vi "Main.vi"(7 "sweep rate, /min":dbl=0.2, 8 "sweep to:":dbl=-0.5, 9 "sweep":T3(radio)=enum."time_sweep") -> ()   [LabVIEW 2017] (continued)
                          tunnel: w368 -> [w372 w376]
                          tunnel: [w372 w374] -> w367
                          frame False {
                            # "not measure SR830 3 out of phase signal (SR830_3_oop)"
                          }
                          frame True {
                            w375 = "SR830_3_oop"
                            # "measure SR830 3 out phase signal (SR830_3_oop)"
                            n376 = local read "SR830 3 addr"() -> (w380:u8)
                            n377 = Number To Decimal String(number=w380) -> (decimal integer string=w381:string)  [unwired: 1 in]
                            n378 = GPIB Clear(3:w381) -> ()  [unwired: 1 in, 2 out]
                            n379 = Build Array (concatenate)(w376, w375) -> (w374:string[])
                            n380 = Concatenate Strings(w379, w375, "\t") -> (w378:string)
                          }
                        }
                        n381 = property on="Figure_axis" class="Arr (strict)"("Value"=w367) -> ()  [unwired: 2 in, 2 out]
                        n382 = property on="data_caption" class="Str"("Value"=w369) -> ()  [unwired: 2 in, 2 out]
                      }
                      frame #6 {
                        # "SR830 4 in phase (SR830_4_ip)"
                        n383 = local read "SR830 4 ip"() -> (w386:bool)
                        n384 = property on="Figure_axis" class="Arr (strict)"() -> ("Value"=w383:string[])  [unwired: 2 in, 2 out]
                        n385 = property on="data_caption" class="Str"() -> ("Value"=w385:string)  [unwired: 2 in, 2 out]
                        n386 = case shown="True" w386 {
                          tunnel: w385 -> [w388 w394]
                          tunnel: [w388 w393] -> w384
                          tunnel: w383 -> [w387 w391]
                          tunnel: [w387 w389] -> w382
                          frame False {
                            # "not measure SR830 4 in phase signal (SR830_4_ip)"
                          }
                          frame True {
                            w390 = "SR830_4_ip"
                            # "measure SR830 4 in phase signal (SR830_4_ip)"
                            n387 = local read "SR830 4 addr"() -> (w395:u8)
                            n388 = Number To Decimal String(number=w395) -> (decimal integer string=w396:string)  [unwired: 1 in]
                            n389 = GPIB Clear(3:w396) -> ()  [unwired: 1 in, 2 out]
                            n390 = Build Array (concatenate)(w391, w390) -> (w389:string[])
                            n391 = Concatenate Strings(w394, w390, "\t") -> (w393:string)
                          }
                        }
                        n392 = property on="Figure_axis" class="Arr (strict)"("Value"=w382) -> ()  [unwired: 2 in, 2 out]
                        n393 = property on="data_caption" class="Str"("Value"=w384) -> ()  [unwired: 2 in, 2 out]
                      }
                      frame #7 {
                        # "SR830 4 out of phase (SR830_4_oop)"
                        n394 = local read "SR830 4 oop"() -> (w401:bool)
                        n395 = property on="Figure_axis" class="Arr (strict)"() -> ("Value"=w398:string[])  [unwired: 2 in, 2 out]
                        n396 = property on="data_caption" class="Str"() -> ("Value"=w400:string)  [unwired: 2 in, 2 out]
                        n397 = case shown="True" w401 {
                          tunnel: w400 -> [w403 w409]
                          tunnel: [w403 w408] -> w399
                          tunnel: w398 -> [w402 w406]
                          tunnel: [w402 w404] -> w397
                          frame False {
                            # "not measure SR830 4 out of phase signal (SR830_4_oop)"
                          }
                          frame True {
                            w405 = "SR830_4_oop"
                            # "measure SR830 4 out of phase signal (SR830_4_oop)"
                            n398 = local read "SR830 4 addr"() -> (w410:u8)
                            n399 = Number To Decimal String(number=w410) -> (decimal integer string=w411:string)  [unwired: 1 in]
                            n400 = GPIB Clear(3:w411) -> ()  [unwired: 1 in, 2 out]
                            n401 = Build Array (concatenate)(w406, w405) -> (w404:string[])
                            n402 = Concatenate Strings(w409, w405, "\t") -> (w408:string)
                          }
                        }
                        n403 = property on="Figure_axis" class="Arr (strict)"("Value"=w397) -> ()  [unwired: 2 in, 2 out]
                        n404 = property on="data_caption" class="Str"("Value"=w399) -> ()  [unwired: 2 in, 2 out]
                      }
                      frame #8 {
                        # "2400 1 voltage measure (2400_1_v)"
                        n405 = local read "2400 1 meas v"() -> (w416:bool)
                        n406 = property on="Figure_axis" class="Arr (strict)"() -> ("Value"=w413:string[])  [unwired: 2 in, 2 out]
                        n407 = property on="data_caption" class="Str"() -> ("Value"=w415:string)  [unwired: 2 in, 2 out]
                        n408 = case shown="True" w416 {
                          tunnel: w415 -> [w418 w424]
                          tunnel: [w418 w423] -> w414
                          tunnel: w413 -> [w417 w421]
                          tunnel: [w417 w419] -> w412
                          frame False {
                            # "not measure 2400 1 voltage (2400_1_v)"
                          }
                          frame True {
                            w420 = "2400_1_v"
                            # "measure 2400 1 voltage (2400_1_v)"
                            n409 = local read "2400 1 addr"() -> (w425:u8)
                            n410 = Number To Decimal String(number=w425) -> (decimal integer string=w426:string)  [unwired: 1 in]
                            n411 = GPIB Clear(3:w426) -> ()  [unwired: 1 in, 2 out]
                            n412 = Build Array (concatenate)(w421, w420) -> (w419:string[])
                            n413 = Concatenate Strings(w424, w420, "\t") -> (w423:string)
                          }
                        }
                        n414 = property on="Figure_axis" class="Arr (strict)"("Value"=w412) -> ()  [unwired: 2 in, 2 out]
                        n415 = property on="data_caption" class="Str"("Value"=w414) -> ()  [unwired: 2 in, 2 out]
                      }
                      frame #9 {
                        # "2400 1 current measure (2400_1_i)"
                        n416 = local read "2400 1 meas i"() -> (w431:bool)
                        n417 = property on="Figure_axis" class="Arr (strict)"() -> ("Value"=w428:string[])  [unwired: 2 in, 2 out]
                        n418 = property on="data_caption" class="Str"() -> ("Value"=w430:string)  [unwired: 2 in, 2 out]
                        n419 = case shown="True" w431 {
                          tunnel: w430 -> [w433 w439]
                          tunnel: [w433 w438] -> w429
                          tunnel: w428 -> [w432 w436]
                          tunnel: [w432 w434] -> w427
                          frame False {
                            # "not measure 2400 1 current (2400_1_i)"
                          }
                          frame True {
                            w435 = "2400_1_i"
                            # "measure 2400 1 current (2400_1_i)"
                            n420 = local read "2400 1 addr"() -> (w440:u8)
                            n421 = Number To Decimal String(number=w440) -> (decimal integer string=w441:string)  [unwired: 1 in]
                            n422 = GPIB Clear(3:w441) -> ()  [unwired: 1 in, 2 out]
                            n423 = Build Array (concatenate)(w436, w435) -> (w434:string[])
                            n424 = Concatenate Strings(w439, w435, "\t") -> (w438:string)
                          }
                        }
                        n425 = property on="Figure_axis" class="Arr (strict)"("Value"=w427) -> ()  [unwired: 2 in, 2 out]
                        n426 = property on="data_caption" class="Str"("Value"=w429) -> ()  [unwired: 2 in, 2 out]
                      }
                      frame #10 {
                        # "2400 2 voltage measure (2400_2_v)"
                        n427 = local read "2400 2 meas v"() -> (w446:bool)
                        n428 = property on="Figure_axis" class="Arr (strict)"() -> ("Value"=w443:string[])  [unwired: 2 in, 2 out]
                        n429 = property on="data_caption" class="Str"() -> ("Value"=w445:string)  [unwired: 2 in, 2 out]
                        n430 = case shown="True" w446 {
                          tunnel: w445 -> [w448 w454]
                          tunnel: [w448 w453] -> w444
                          tunnel: w443 -> [w447 w451]
                          tunnel: [w447 w449] -> w442
                          frame False {
                            # "not measure 2400 2 voltage (2400_2_v)"
                          }
                          frame True {
                            w450 = "2400_2_v"
                            # "measure 2400 2 voltage (2400_2_v)"
                            n431 = local read "2400 2 addr"() -> (w455:u8)
                            n432 = Number To Decimal String(number=w455) -> (decimal integer string=w456:string)  [unwired: 1 in]
                            n433 = GPIB Clear(3:w456) -> ()  [unwired: 1 in, 2 out]
                            n434 = Build Array (concatenate)(w451, w450) -> (w449:string[])
                            n435 = Concatenate Strings(w454, w450, "\t") -> (w453:string)
                          }
                        }
                        n436 = property on="Figure_axis" class="Arr (strict)"("Value"=w442) -> ()  [unwired: 2 in, 2 out]
                        n437 = property on="data_caption" class="Str"("Value"=w444) -> ()  [unwired: 2 in, 2 out]
                      }
                      frame #11 {
                        # "2400 2 current measure (2400_2_i)"
                        n438 = local read "2400 2 meas i"() -> (w461:bool)
                        n439 = property on="Figure_axis" class="Arr (strict)"() -> ("Value"=w458:string[])  [unwired: 2 in, 2 out]
                        n440 = property on="data_caption" class="Str"() -> ("Value"=w460:string)  [unwired: 2 in, 2 out]
                        n441 = case shown="True" w461 {
                          tunnel: w460 -> [w463 w469]
                          tunnel: [w463 w468] -> w459
                          tunnel: w458 -> [w462 w466]
                          tunnel: [w462 w464] -> w457
                          frame False {
                            # "not measure 2400 2 current (2400_2_i)"
                          }
                          frame True {
                            w465 = "2400_2_i"
                            # "measure 2400 2 current (2400_2_i)"
                            n442 = local read "2400 2 addr"() -> (w470:u8)
                            n443 = Number To Decimal String(number=w470) -> (decimal integer string=w471:string)  [unwired: 1 in]
                            n444 = GPIB Clear(3:w471) -> ()  [unwired: 1 in, 2 out]
                            n445 = Build Array (concatenate)(w466, w465) -> (w464:string[])
                            n446 = Concatenate Strings(w469, w465, "\t") -> (w468:string)
                          }
                        }
                        n447 = property on="Figure_axis" class="Arr (strict)"("Value"=w457) -> ()  [unwired: 2 in, 2 out]
                        n448 = property on="data_caption" class="Str"("Value"=w459) -> ()  [unwired: 2 in, 2 out]
                      }
                      frame #12 {
                        # "2400 3 voltage measure (2400_3_v)"
                        n449 = local read "2400 3 meas v"() -> (w476:bool)
                        n450 = property on="Figure_axis" class="Arr (strict)"() -> ("Value"=w473:string[])  [unwired: 2 in, 2 out]
                        n451 = property on="data_caption" class="Str"() -> ("Value"=w475:string)  [unwired: 2 in, 2 out]
                        n452 = case shown="True" w476 {
                          tunnel: w475 -> [w478 w484]
                          tunnel: [w478 w483] -> w474
                          tunnel: w473 -> [w477 w481]
                          tunnel: [w477 w479] -> w472
                          frame False {
                            # "not measure 2400 3 voltage (2400_3_v)"
                          }
                          frame True {
                            w480 = "2400_3_v"
                            # "measure 2400 3 voltage (2400_3_v)"
                            n453 = local read "2400 3 addr"() -> (w485:u8)
                            n454 = Number To Decimal String(number=w485) -> (decimal integer string=w486:string)  [unwired: 1 in]
                            n455 = GPIB Clear(3:w486) -> ()  [unwired: 1 in, 2 out]
                            n456 = Build Array (concatenate)(w481, w480) -> (w479:string[])
                            n457 = Concatenate Strings(w484, w480, "\t") -> (w483:string)
                          }
                        }
                        n458 = property on="Figure_axis" class="Arr (strict)"("Value"=w472) -> ()  [unwired: 2 in, 2 out]
                        n459 = property on="data_caption" class="Str"("Value"=w474) -> ()  [unwired: 2 in, 2 out]
                      }
                      frame #13 {
                        # "2400 3 current measure (2400_3_i)"
                        n460 = local read "2400 3 meas i"() -> (w491:bool)
                        n461 = property on="Figure_axis" class="Arr (strict)"() -> ("Value"=w488:string[])  [unwired: 2 in, 2 out]
                        n462 = property on="data_caption" class="Str"() -> ("Value"=w490:string)  [unwired: 2 in, 2 out]
                        n463 = case shown="True" w491 {
                          tunnel: w490 -> [w493 w499]
                          tunnel: [w493 w498] -> w489
                          tunnel: w488 -> [w492 w496]
                          tunnel: [w492 w494] -> w487
                          frame False {
                            # "not measure 2400 3 current (2400_3_i)"
                          }
                          frame True {
                            w495 = "2400_3_i"
                            # "measure 2400 3 current (2400_3_i)"
                            n464 = local read "2400 3 addr"() -> (w500:u8)
                            n465 = Number To Decimal String(number=w500) -> (decimal integer string=w501:string)  [unwired: 1 in]
                            n466 = GPIB Clear(3:w501) -> ()  [unwired: 1 in, 2 out]
                            n467 = Build Array (concatenate)(w496, w495) -> (w494:string[])
                            n468 = Concatenate Strings(w499, w495, "\t") -> (w498:string)
                          }
                        }
                        n469 = property on="Figure_axis" class="Arr (strict)"("Value"=w487) -> ()  [unwired: 2 in, 2 out]
                        n470 = property on="data_caption" class="Str"("Value"=w489) -> ()  [unwired: 2 in, 2 out]
                      }
                      frame #14 {
                        # "2182A 1 channel 1 measure (2182A_1_ch1)"
                        n471 = local read "2182A 1 ch1"() -> (w506:bool)
                        n472 = property on="Figure_axis" class="Arr (strict)"() -> ("Value"=w503:string[])  [unwired: 2 in, 2 out]
                        n473 = property on="data_caption" class="Str"() -> ("Value"=w505:string)  [unwired: 2 in, 2 out]
                        n474 = case shown="False" w506 {
                          tunnel: w505 -> [w508 w514]
                          tunnel: [w508 w513] -> w504
                          tunnel: w503 -> [w507 w511]
                          tunnel: [w507 w509] -> w502
                          frame False {
                            # "not measure 2182A 1 channel 1 (2182A_1_ch1)"
                          }
                          frame True {
                            w510 = "2182A_1_ch1"
                            # "measure 2182A 1 channel 1 (2182A_1_ch1)"
                            n475 = local read "2182A 1 addr"() -> (w515:u8)
                            n476 = Number To Decimal String(number=w515) -> (decimal integer string=w516:string)  [unwired: 1 in]
                            n477 = GPIB Clear(3:w516) -> ()  [unwired: 1 in, 2 out]
                            n478 = Build Array (concatenate)(w511, w510) -> (w509:string[])
                            n479 = Concatenate Strings(w514, w510, "\t") -> (w513:string)
                          }
                        }
                        n480 = property on="Figure_axis" class="Arr (strict)"("Value"=w502) -> ()  [unwired: 2 in, 2 out]
                        n481 = property on="data_caption" class="Str"("Value"=w504) -> ()  [unwired: 2 in, 2 out]
                      }
                      frame #15 {
                        # "2182A 1 channel 2 measure (2182A_1_ch2)"
                        n482 = local read "2182A 1 ch2"() -> (w521:bool)
                        n483 = property on="Figure_axis" class="Arr (strict)"() -> ("Value"=w518:string[])  [unwired: 2 in, 2 out]
                        n484 = property on="data_caption" class="Str"() -> ("Value"=w520:string)  [unwired: 2 in, 2 out]
                        n485 = case shown="True" w521 {
                          tunnel: w520 -> [w523 w529]
                          tunnel: [w523 w528] -> w519
                          tunnel: w518 -> [w522 w526]
                          tunnel: [w522 w524] -> w517
                          frame False {
                            # "not measure 2182A 1 channel 2 (2182A_1_ch2)"
                          }
                          frame True {
                            w525 = "2182A_1_ch2"
                            # "measure 2182A 1 channel 2 (2182A_1_ch2)"
                            n486 = local read "2182A 1 addr"() -> (w530:u8)
                            n487 = Number To Decimal String(number=w530) -> (decimal integer string=w531:string)  [unwired: 1 in]
                            n488 = GPIB Clear(3:w531) -> ()  [unwired: 1 in, 2 out]
                            n489 = Build Array (concatenate)(w526, w525) -> (w524:string[])
                            n490 = Concatenate Strings(w529, w525, "\t") -> (w528:string)
                          }
                        }
                        n491 = property on="Figure_axis" class="Arr (strict)"("Value"=w517) -> ()  [unwired: 2 in, 2 out]
                        n492 = property on="data_caption" class="Str"("Value"=w519) -> ()  [unwired: 2 in, 2 out]
                      }
                      frame #16 {
                        # "2182A 2 channel 1 measure (2182A_2_ch1)"
                        n493 = local read "2182A 2 ch1"() -> (w536:bool)
                        n494 = property on="Figure_axis" class="Arr (strict)"() -> ("Value"=w533:string[])  [unwired: 2 in, 2 out]
                        n495 = property on="data_caption" class="Str"() -> ("Value"=w535:string)  [unwired: 2 in, 2 out]
                        n496 = case shown="True" w536 {
                          tunnel: w535 -> [w538 w544]
                          tunnel: [w538 w543] -> w534
                          tunnel: w533 -> [w537 w541]
                          tunnel: [w537 w539] -> w532
                          frame False {
                            # "not measure 2182A 2 channel 1 (2182A_2_ch1)"
                          }
                          frame True {
                            w540 = "2182A_2_ch1"
                            # "measure 2182A 2 channel 1 (2182A_2_ch1)"
                            n497 = local read "2182A 2 addr"() -> (w545:u8)
                            n498 = Number To Decimal String(number=w545) -> (decimal integer string=w546:string)  [unwired: 1 in]
                            n499 = GPIB Clear(3:w546) -> ()  [unwired: 1 in, 2 out]
                            n500 = Build Array (concatenate)(w541, w540) -> (w539:string[])
                            n501 = Concatenate Strings(w544, w540, "\t") -> (w543:string)
                          }
                        }
                        n502 = property on="Figure_axis" class="Arr (strict)"("Value"=w532) -> ()  [unwired: 2 in, 2 out]
                        n503 = property on="data_caption" class="Str"("Value"=w534) -> ()  [unwired: 2 in, 2 out]
                      }
                      frame #17 {
                        # "2182A 2 channel 2 measure (2182A_2_ch2)"
                        n504 = local read "2182A 2 ch2"() -> (w551:bool)
                        n505 = property on="Figure_axis" class="Arr (strict)"() -> ("Value"=w548:string[])  [unwired: 2 in, 2 out]
                        n506 = property on="data_caption" class="Str"() -> ("Value"=w550:string)  [unwired: 2 in, 2 out]
                        n507 = case shown="True" w551 {
                          tunnel: w550 -> [w553 w559]
                          tunnel: [w553 w558] -> w549
                          tunnel: w548 -> [w552 w556]
                          tunnel: [w552 w554] -> w547
                          frame False {
                            # "not measure 2182A 2 channel 2 (2182A_2_ch2)"
                          }
                          frame True {
                            w555 = "2182A_2_ch2"
                            # "measure 2182A 2 channel 2 (2182A_2_ch2)"
                            n508 = local read "2182A 2 addr"() -> (w560:u8)
                            n509 = Number To Decimal String(number=w560) -> (decimal integer string=w561:string)  [unwired: 1 in]
                            n510 = GPIB Clear(3:w561) -> ()  [unwired: 1 in, 2 out]
                            n511 = Build Array (concatenate)(w556, w555) -> (w554:string[])
                            n512 = Concatenate Strings(w559, w555, "\t") -> (w558:string)
                          }
                        }
                        n513 = property on="Figure_axis" class="Arr (strict)"("Value"=w547) -> ()  [unwired: 2 in, 2 out]
                        n514 = property on="data_caption" class="Str"("Value"=w549) -> ()  [unwired: 2 in, 2 out]
                      }
                      frame #18 {
                        # "2182A 3 channel 1 measure (2182A_3_ch1)"
                        n515 = local read "2182A 3 ch1"() -> (w566:bool)
                        n516 = property on="Figure_axis" class="Arr (strict)"() -> ("Value"=w563:string[])  [unwired: 2 in, 2 out]
                        n517 = property on="data_caption" class="Str"() -> ("Value"=w565:string)  [unwired: 2 in, 2 out]
                        n518 = case shown="True" w566 {
                          tunnel: w565 -> [w568 w574]
                          tunnel: [w568 w573] -> w564
                          tunnel: w563 -> [w567 w571]
                          tunnel: [w567 w569] -> w562
                          frame False {
                            # "not measure 2182A 3 channel 1 (2182A_3_ch1)"
                          }
                          frame True {
                            w570 = "2182A_3_ch1"
                            # "measure 2182A 3 channel 1 (2182A_3_ch1)"
                            n519 = local read "2182A 3 addr"() -> (w575:u8)
                            n520 = Number To Decimal String(number=w575) -> (decimal integer string=w576:string)  [unwired: 1 in]
                            n521 = GPIB Clear(3:w576) -> ()  [unwired: 1 in, 2 out]
                            n522 = Build Array (concatenate)(w571, w570) -> (w569:string[])
                            n523 = Concatenate Strings(w574, w570, "\t") -> (w573:string)
                          }
                        }
                        n524 = property on="Figure_axis" class="Arr (strict)"("Value"=w562) -> ()  [unwired: 2 in, 2 out]
                        n525 = property on="data_caption" class="Str"("Value"=w564) -> ()  [unwired: 2 in, 2 out]
                      }
                      frame #19 {
                        # "2182A 3 channel 2 measure (2182A_3_ch2)"
                        n526 = local read "2182A 3 ch2"() -> (w581:bool)
                        n527 = property on="Figure_axis" class="Arr (strict)"() -> ("Value"=w578:string[])  [unwired: 2 in, 2 out]
                        n528 = property on="data_caption" class="Str"() -> ("Value"=w580:string)  [unwired: 2 in, 2 out]
                        n529 = case shown="False" w581 {
                          tunnel: w580 -> [w583 w589]
                          tunnel: [w583 w588] -> w579
                          tunnel: w578 -> [w582 w586]
                          tunnel: [w582 w584] -> w577
                          frame False {
                            # "not measure 2182A 3 channel 2 (2182A_3_ch2)"
                          }
                          frame True {
                            w585 = "2182A_3_ch2"
                            # "measure 2182A 3 channel 2 (2182A_3_ch2)"
                            n530 = local read "2182A 3 addr"() -> (w590:u8)
                            n531 = Number To Decimal String(number=w590) -> (decimal integer string=w591:string)  [unwired: 1 in]
                            n532 = GPIB Clear(3:w591) -> ()  [unwired: 1 in, 2 out]
                            n533 = Build Array (concatenate)(w586, w585) -> (w584:string[])
                            n534 = Concatenate Strings(w589, w585, "\t") -> (w588:string)
                          }
                        }
                        n535 = property on="Figure_axis" class="Arr (strict)"("Value"=w577) -> ()  [unwired: 2 in, 2 out]
                        n536 = property on="data_caption" class="Str"("Value"=w579) -> ()  [unwired: 2 in, 2 out]
                      }
                      frame #20 {
                        # "2182A 4 channel 1 measure (2182A_4_ch1)"
                        n537 = local read "2182A 4 ch1"() -> (w596:bool)
                        n538 = property on="Figure_axis" class="Arr (strict)"() -> ("Value"=w593:string[])  [unwired: 2 in, 2 out]
                        n539 = property on="data_caption" class="Str"() -> ("Value"=w595:string)  [unwired: 2 in, 2 out]
                        n540 = case shown="True" w596 {
                          tunnel: w595 -> [w598 w604]
                          tunnel: [w598 w603] -> w594
                          tunnel: w593 -> [w597 w601]
                          tunnel: [w597 w599] -> w592
                          frame False {
                            # "not measure 2182A 4 channel 1 (2182A_4_ch1)"
                          }
                          frame True {
                            w600 = "2182A_4_ch1"
                            # "measure 2182A 4 channel 1 (2182A_4_ch1)"
                            n541 = local read "2182A 4 addr"() -> (w605:u8)
                            n542 = Number To Decimal String(number=w605) -> (decimal integer string=w606:string)  [unwired: 1 in]
                            n543 = GPIB Clear(3:w606) -> ()  [unwired: 1 in, 2 out]
                            n544 = Build Array (concatenate)(w601, w600) -> (w599:string[])
                            n545 = Concatenate Strings(w604, w600, "\t") -> (w603:string)
                          }
                        }
                        n546 = property on="Figure_axis" class="Arr (strict)"("Value"=w592) -> ()  [unwired: 2 in, 2 out]
                        n547 = property on="data_caption" class="Str"("Value"=w594) -> ()  [unwired: 2 in, 2 out]
                      }
                      frame #21 {
                        # "2182A 4 channel 2 measure (2182A_4_ch2)"
                        n548 = local read "2182A 4 ch2"() -> (w611:bool)
                        n549 = property on="Figure_axis" class="Arr (strict)"() -> ("Value"=w608:string[])  [unwired: 2 in, 2 out]
                        n550 = property on="data_caption" class="Str"() -> ("Value"=w610:string)  [unwired: 2 in, 2 out]
                        n551 = case shown="True" w611 {
                          tunnel: w610 -> [w613 w619]
                          tunnel: [w613 w618] -> w609
                          tunnel: w608 -> [w612 w616]
                          tunnel: [w612 w614] -> w607
                          frame False {
                            # "not measure 2182A 4 channel 2 (2182A_4_ch2)"
                          }
                          frame True {
                            w615 = "2182A_4_ch2"
                            # "measure 2182A 4 channel 2 (2182A_4_ch2)"
                            n552 = local read "2182A 4 addr"() -> (w620:u8)
                            n553 = Number To Decimal String(number=w620) -> (decimal integer string=w621:string)  [unwired: 1 in]
                            n554 = GPIB Clear(3:w621) -> ()  [unwired: 1 in, 2 out]
                            n555 = Build Array (concatenate)(w616, w615) -> (w614:string[])
                            n556 = Concatenate Strings(w619, w615, "\t") -> (w618:string)
                          }
                        }
                        n557 = property on="Figure_axis" class="Arr (strict)"("Value"=w607) -> ()  [unwired: 2 in, 2 out]
                        n558 = property on="data_caption" class="Str"("Value"=w609) -> ()  [unwired: 2 in, 2 out]
                      }
                      frame #22 {
                        # "2636A smua measure voltage (2636A_smua_v)"
                        n559 = local read "2636A smua meas v"() -> (w626:bool)
                        n560 = property on="Figure_axis" class="Arr (strict)"() -> ("Value"=w623:string[])  [unwired: 2 in, 2 out]
                        n561 = property on="data_caption" class="Str"() -> ("Value"=w625:string)  [unwired: 2 in, 2 out]
                        n562 = case shown="True" w626 {
                          tunnel: w625 -> [w628 w639]
                          tunnel: [w628 w638] -> w624
                          tunnel: w623 -> [w627 w636]
                          tunnel: [w627 w634] -> w622
                          frame False {
                            # "not measure voltage on 2636A smua (2636A_smua_v)"
                          }
                          frame True {
                            w635 = "2636A_smua_v"
                            # "measure voltage on 2636A smua (2636A_smua_v)"
                            n563 = local read "2336A addr"() -> (w630:refnum<visa-resource-name>)
                            n564 = VISA Open(VISA resource name=w630) -> (VISA resource name=w629:refnum<visa-resource-name>, error out=w631:errorcluster)  [unwired: 4 in]
                            n565 = VISA Clear(VISA resource name=w629, error in (no error)=w631) -> (VISA resource name out=w633:refnum<visa-resource-name>)  [unwired: 1 out]
                            n566 = property class="Instr"(reference=w633, "General Settings:Timeout Value"=u32 10000) -> ()  [unwired: 1 in, 2 out]
                            n567 = Build Array (concatenate)(w636, w635) -> (w634:string[])
                            n568 = Concatenate Strings(w639, w635, "\t") -> (w638:string)
                          }
                        }
                        n569 = property on="Figure_axis" class="Arr (strict)"("Value"=w622) -> ()  [unwired: 2 in, 2 out]
                        n570 = property on="data_caption" class="Str"("Value"=w624) -> ()  [unwired: 2 in, 2 out]
                      }
                      frame #23 {
                        # "2636A smua measure current (2636A_smua_i)"
                        n571 = local read "2636A smua meas i"() -> (w644:bool)
                        n572 = property on="Figure_axis" class="Arr (strict)"() -> ("Value"=w641:string[])  [unwired: 2 in, 2 out]
                        n573 = property on="data_caption" class="Str"() -> ("Value"=w643:string)  [unwired: 2 in, 2 out]
                        n574 = case shown="True" w644 {
                          tunnel: w643 -> [w646 w657]
                          tunnel: [w646 w656] -> w642
                          tunnel: w641 -> [w645 w654]
                          tunnel: [w645 w652] -> w640
                          frame False {
                            # "not measure current on 2636A smua (2636A_smua_i)"
                          }
                          frame True {
                            w653 = "2636A_smua_i"
                            # "measure current on 2636A smua (2636A_smua_i)"
                            n575 = local read "2336A addr"() -> (w649:refnum<visa-resource-name>)
                            n576 = VISA Open(VISA resource name=w649) -> (VISA resource name=w648:refnum<visa-resource-name>, error out=w647:errorcluster)  [unwired: 4 in]
                            n577 = VISA Clear(VISA resource name=w648, error in (no error)=w647) -> (VISA resource name out=w650:refnum<visa-resource-name>)  [unwired: 1 out]
                            n578 = Build Array (concatenate)(w654, w653) -> (w652:string[])
                            n579 = property class="Instr"(reference=w650, "General Settings:Timeout Value"=u32 10000) -> ()  [unwired: 1 in, 2 out]
                            n580 = Concatenate Strings(w657, w653, "\t") -> (w656:string)
                          }
                        }
                        n581 = property on="Figure_axis" class="Arr (strict)"("Value"=w640) -> ()  [unwired: 2 in, 2 out]
                        n582 = property on="data_caption" class="Str"("Value"=w642) -> ()  [unwired: 2 in, 2 out]
                      }
                      frame #24 {
                        # "2636A smub measure voltage (2636A_smub_v)"
                        n583 = local read "2636A smub meas v"() -> (w662:bool)
                        n584 = property on="Figure_axis" class="Arr (strict)"() -> ("Value"=w659:string[])  [unwired: 2 in, 2 out]
                        n585 = property on="data_caption" class="Str"() -> ("Value"=w661:string)  [unwired: 2 in, 2 out]
                        n586 = case shown="True" w662 {
                          tunnel: w661 -> [w664 w675]
                          tunnel: [w664 w674] -> w660
                          tunnel: w659 -> [w663 w672]
                          tunnel: [w663 w670] -> w658
                          frame False {
                            # "not measure voltage on 2636A smub (2636A_smub_v)"
                          }
                          frame True {
                            w671 = "2636A_smub_v"
                            # "measure voltage on 2636A smub (2636A_smub_v)"
                            n587 = local read "2336A addr"() -> (w666:refnum<visa-resource-name>)
                            n588 = VISA Open(VISA resource name=w666) -> (VISA resource name=w665:refnum<visa-resource-name>, error out=w667:errorcluster)  [unwired: 4 in]
                            n589 = VISA Clear(VISA resource name=w665, error in (no error)=w667) -> (VISA resource name out=w668:refnum<visa-resource-name>)  [unwired: 1 out]
                            n590 = Build Array (concatenate)(w672, w671) -> (w670:string[])
                            n591 = property class="Instr"(reference=w668, "General Settings:Timeout Value"=u32 10000) -> ()  [unwired: 1 in, 2 out]
                            n592 = Concatenate Strings(w675, w671, "\t") -> (w674:string)
                          }
                        }
                        n593 = property on="Figure_axis" class="Arr (strict)"("Value"=w658) -> ()  [unwired: 2 in, 2 out]
                        n594 = property on="data_caption" class="Str"("Value"=w660) -> ()  [unwired: 2 in, 2 out]
                      }
                      frame #25 {
                        # "2636A smub measure current (2636A_smub_i)"
                        n595 = local read "2636A smub meas i"() -> (w680:bool)
                        n596 = property on="Figure_axis" class="Arr (strict)"() -> ("Value"=w677:string[])  [unwired: 2 in, 2 out]
                        n597 = property on="data_caption" class="Str"() -> ("Value"=w679:string)  [unwired: 2 in, 2 out]
                        n598 = case shown="True" w680 {
                          tunnel: w679 -> [w682 w693]
                          tunnel: [w682 w692] -> w678
                          tunnel: w677 -> [w681 w690]
                          tunnel: [w681 w688] -> w676
                          frame False {
                            # "not measure current on 2636A smub (2636A_smub_i)"
                          }
                          frame True {
                            w689 = "2636A_smub_i"
                            # "measure current on 2636A smub (2636A_smub_i)"
                            n599 = local read "2336A addr"() -> (w683:refnum<visa-resource-name>)
                            n600 = VISA Open(VISA resource name=w683) -> (VISA resource name=w684:refnum<visa-resource-name>, error out=w685:errorcluster)  [unwired: 4 in]
                            n601 = VISA Clear(VISA resource name=w684, error in (no error)=w685) -> (VISA resource name out=w686:refnum<visa-resource-name>)  [unwired: 1 out]
                            n602 = Build Array (concatenate)(w690, w689) -> (w688:string[])
                            n603 = property class="Instr"(reference=w686, "General Settings:Timeout Value"=u32 10000) -> ()  [unwired: 1 in, 2 out]
                            n604 = Concatenate Strings(w693, w689, "\t") -> (w692:string)
                          }
                        }
                        n605 = property on="Figure_axis" class="Arr (strict)"("Value"=w676) -> ()  [unwired: 2 in, 2 out]
                        n606 = property on="data_caption" class="Str"("Value"=w678) -> ()  [unwired: 2 in, 2 out]
                      }
                      frame #26 {
                        # "measure time"
                        n607 = local read "measure time"() -> (w698:bool)
                        n608 = property on="Figure_axis" class="Arr (strict)"() -> ("Value"=w695:string[])  [unwired: 2 in, 2 out]
                        n609 = property on="data_caption" class="Str"() -> ("Value"=w697:string)  [unwired: 2 in, 2 out]
                        n610 = case shown="True" w698 {
                          tunnel: w697 -> [w700 w706]
                          tunnel: [w700 w705] -> w696
                          tunnel: w695 -> [w699 w703]
                          tunnel: [w699 w701] -> w694
                          frame False {
                            # "not measuring time"
                          }
                          frame True {
                            w702 = "time"
                            # "measuring time"
                            n611 = Build Array (concatenate)(w703, w702) -> (w701:string[])
                            n612 = Concatenate Strings(w706, w702, "\t") -> (w705:string)
                          }
                        }
                        n613 = property on="Figure_axis" class="Arr (strict)"("Value"=w694) -> ()  [unwired: 2 in, 2 out]
                        n614 = property on="data_caption" class="Str"("Value"=w696) -> ()  [unwired: 2 in, 2 out]
                      }
                      frame #27 {
                        # "Measure magnetic field on Teslatron_iPS"
                        n615 = local read "iPS_MagnetField"() -> (w711:bool)
                        n616 = property on="Figure_axis" class="Arr (strict)"() -> ("Value"=w708:string[])  [unwired: 2 in, 2 out]
                        n617 = property on="data_caption" class="Str"() -> ("Value"=w710:string)  [unwired: 2 in, 2 out]
                        n618 = case shown="True" w711 {
                          tunnel: w710 -> [w713 w719]
                          tunnel: [w713 w718] -> w709
                          tunnel: w708 -> [w712 w716]
                          tunnel: [w712 w714] -> w707
                          frame False {
                            # "do not Measure magnetic field on IPS120-0"
                          }
                          frame True {
                            w715 = "iPS_MagnetField"
                            # "Measure magnetic field on Teslatron_iPS_Field"
                            n619 = Build Array (concatenate)(w716, w715) -> (w714:string[])
                            n620 = Concatenate Strings(w719, w715, "\t") -> (w718:string)
                          }
                        }
                        n621 = property on="Figure_axis" class="Arr (strict)"("Value"=w707) -> ()  [unwired: 2 in, 2 out]
                        n622 = property on="data_caption" class="Str"("Value"=w709) -> ()  [unwired: 2 in, 2 out]
                      }
                      frame #28 {
                        # "Measure magnetic field on Teslatron_iPS"
                        n623 = property on="iTC_Sample_T" class="Bool (strict)"() -> ("Value"=w720:bool)  [unwired: 2 in, 2 out]
                        n624 = property on="Figure_axis" class="Arr (strict)"() -> ("Value"=w722:string[])  [unwired: 2 in, 2 out]
                        n625 = property on="data_caption" class="Str"() -> ("Value"=w724:string)  [unwired: 2 in, 2 out]
                        n626 = case shown="True" w720 {
                          tunnel: w724 -> [w726 w732]
                          tunnel: [w726 w731] -> w723
                          tunnel: w722 -> [w725 w729]
                          tunnel: [w725 w727] -> w721
                          frame False {
                            # "not measure 2461 voltage (2461_meas_v)"
                          }
                          frame True {
                            w728 = "iTC_sample_T"
                            n627 = Build Array (concatenate)(w729, w728) -> (w727:string[])
                            n628 = Concatenate Strings(w732, w728, "\t") -> (w731:string)
                          }
                        }
                        n629 = property on="Figure_axis" class="Arr (strict)"("Value"=w721) -> ()  [unwired: 2 in, 2 out]
                        n630 = property on="data_caption" class="Str"("Value"=w723) -> ()  [unwired: 2 in, 2 out]
                      }
                      frame #29 {
                        # "Measure magnetic field on Teslatron_iPS"
                        n631 = property on="CH_A" class="Bool (strict)"() -> ("Value"=w733:bool)  [unwired: 2 in, 2 out]
                        n632 = property on="Figure_axis" class="Arr (strict)"() -> ("Value"=w735:string[])  [unwired: 2 in, 2 out]
                        n633 = property on="data_caption" class="Str"() -> ("Value"=w737:string)  [unwired: 2 in, 2 out]
                        n634 = case shown="True" w733 {
                          tunnel: w737 -> [w739 w745]
                          tunnel: [w739 w744] -> w736
                          tunnel: w735 -> [w738 w742]
                          tunnel: [w738 w740] -> w734
                          frame False {
                            # "not measure 2461 voltage (2461_meas_v)"
                          }
                          frame True {
                            w741 = "iTC_CH_A"
                            n635 = Build Array (concatenate)(w742, w741) -> (w740:string[])
                            n636 = Concatenate Strings(w745, w741, "\t") -> (w744:string)
                          }
                        }
                        n637 = property on="Figure_axis" class="Arr (strict)"("Value"=w734) -> ()  [unwired: 2 in, 2 out]
                        n638 = property on="data_caption" class="Str"("Value"=w736) -> ()  [unwired: 2 in, 2 out]
                      }
                      frame #30 {
                        # "Measure magnetic field on Teslatron_iPS"
                        n639 = property on="CH_B" class="Bool (strict)"() -> ("Value"=w746:bool)  [unwired: 2 in, 2 out]
                        n640 = property on="Figure_axis" class="Arr (strict)"() -> ("Value"=w748:string[])  [unwired: 2 in, 2 out]
                        n641 = property on="data_caption" class="Str"() -> ("Value"=w750:string)  [unwired: 2 in, 2 out]
                        n642 = case shown="True" w746 {
                          tunnel: w750 -> [w752 w758]
                          tunnel: [w752 w757] -> w749
                          tunnel: w748 -> [w751 w755]
                          tunnel: [w751 w753] -> w747
                          frame False {
                            # "not measure 2461 voltage (2461_meas_v)"
                          }
                          frame True {
                            w754 = "iTC_CH_B"
                            n643 = Build Array (concatenate)(w755, w754) -> (w753:string[])
                            n644 = Concatenate Strings(w758, w754, "\t") -> (w757:string)
                          }
                        }
                        n645 = property on="Figure_axis" class="Arr (strict)"("Value"=w747) -> ()  [unwired: 2 in, 2 out]
                        n646 = property on="data_caption" class="Str"("Value"=w749) -> ()  [unwired: 2 in, 2 out]
                      }
                    }
                  }
                  frame #2 {
                    # "0 = SR830_1_ip\n1 = SR830_1_oop\n2 = SR830_2_ip\n3 = SR830_2_oop\n4 = SR830_3_ip\n5 = SR830_3_oop\n6 = SR830_4_ip \n7 = SR830_4_oop \n8= 2400_1_v \n9 = 2400_1_i \n10 = 2400_2_v\n11 = 2400_2_i \n12 = 2400_3_v \n13 = 2400_3_i \n14 = 2182A_1_ch1 \n15 = 2182A_1_ch2 \n16 = 2182A_2_ch1 \n17 = 2182A_2_ch2\n18 = 2182A_3_ch1 \n19 = 2182A_3_ch2 \n20 = 2182A_4_ch1 \n21 = 2182A_4_ch2 \n22 = 2636A_smua_v \n23 = 2636A_smua_i \n24 = 2636A_smub_v \n25 = 2636A_smub_i \n26 = time\n27 = iPS_120\n28 = iTC _sample_T\n29= iTC _CH_A\n30=iTC_CH_B\n31 = Step_Value"
                    n647 = stacked-sequence {
                      frame #0 {
                        w763 = dbl[] []  # Empty array for data
                        # "clear data array before each measurement cycle"
                        n648 = property on="data" class="Arr (strict)"("Value"=w763) -> (error out=w762:errorcluster)  [unwired: 2 in, 1 out]
                        n649 = property on="Sweep Channel" class="DigNum (strict)"() -> ("Value"=w759:dbl)  [unwired: 2 in, 2 out]
                        n650 = property on="data" class="Arr (strict)"(error in=w762) -> ("Value"=w761:dbl[])  [unwired: 1 in, 2 out]
                        n651 = Build Array (concatenate)(w761, w759) -> (w760:dbl[])
                        n652 = property on="data" class="Arr (strict)"("Value"=w760) -> ()  [unwired: 2 in, 2 out]
                      }
                      frame #1 {
                        n653 = stacked-sequence "measurement sequence" {
                          frame #0 {
                            # "check if in-phase\nsignal on lock-in 1 \nis to be measured"
                            n654 = property on="data" class="Arr (strict)"() -> ("Value"=w765:dbl[])  [unwired: 2 in, 2 out]
                            n655 = local read "SR830 1 ip"() -> (w764:bool)
                            n656 = case shown="True" w764 {
                              tunnel: w765 -> [w767 w776]
                              tunnel: [w767 w775] -> w766
                              frame False {
                                # "we are not measuring in phase signal on lock-in 1 (SR830_1_ip)"
                              }
                              frame True {
                                # "we are  measuring lock-in 1, in phase (SR830_1_ip)"
                                n657 = local read "SR830 1 addr"() -> (w769:u8)
                                n658 = Number To Decimal String(number=w769) -> (decimal integer string=w768:string)  [unwired: 1 in]
                                n659 = GPIB Write(0:w768, 1:"OUTR?1") -> (6:w774:errorcluster)  [unwired: 3 in, 1 out]
                                n660 = GPIB Read(0:w768, 1:3200, 3:w774) -> (5:w772:string)  [unwired: 2 in, 2 out]
                                n661 = Fract/Exp String To Number(string=w772) -> (number=w771:dbl)  [unwired: 3 in, 1 out]
                                n662 = Build Array (concatenate)(w776, w771) -> (w775:dbl[])
                              }
                            }
                            n663 = property on="data" class="Arr (strict)"("Value"=w766) -> ()  [unwired: 2 in, 2 out]
                          }
                          frame #1 {
                            # "check if out-of-phase\nsignal on lock-in 1 \nis to be measured"
                            n664 = property on="data" class="Arr (strict)"() -> ("Value"=w778:dbl[])  [unwired: 2 in, 2 out]
                            n665 = local read "SR830 1 oop"() -> (w777:bool)
                            n666 = case shown="True" w777 {
                              tunnel: w778 -> [w780 w789]
                              tunnel: [w780 w788] -> w779
                              frame False {
                                # "we are not measuring out of phase signal on lock-in 1 (SR830_1_oop)"
                              }
                              frame True {
                                # "we are  measuring lock-in 1, out of phase (SR830_1_oop)"
                                n667 = local read "SR830 1 addr"() -> (w782:u8)
                                n668 = Number To Decimal String(number=w782) -> (decimal integer string=w781:string)  [unwired: 1 in]
                                n669 = GPIB Write(0:w781, 1:"OUTR?2") -> (6:w787:errorcluster)  [unwired: 3 in, 1 out]
                                n670 = GPIB Read(0:w781, 1:3200, 3:w787) -> (5:w785:string)  [unwired: 2 in, 2 out]
                                n671 = Fract/Exp String To Number(string=w785) -> (number=w784:dbl)  [unwired: 3 in, 1 out]
                                n672 = Build Array (concatenate)(w789, w784) -> (w788:dbl[])
                              }
                            }
                            n673 = property on="data" class="Arr (strict)"("Value"=w779) -> ()  [unwired: 2 in, 2 out]
                          }
                          frame #2 {
                            # "check if in-phase\nsignal on lock-in 2 \nis to be measured"
                            n674 = property on="data" class="Arr (strict)"() -> ("Value"=w791:dbl[])  [unwired: 2 in, 2 out]
                            n675 = local read "SR830 2 ip"() -> (w790:bool)
                            n676 = case shown="True" w790 {
                              tunnel: w791 -> [w793 w802]
                              tunnel: [w793 w801] -> w792
                              frame False {
                                # "we are not measuring in phase signal on lock-in 2 (SR830_2_ip)"
                              }
                              frame True {
                                # "we are  measuring lock-in 2, in phase (SR830_2_ip)"
                                n677 = local read "SR830 2 addr"() -> (w795:u8)
                                n678 = Number To Decimal String(number=w795) -> (decimal integer string=w794:string)  [unwired: 1 in]
                                n679 = GPIB Write(0:w794, 1:"OUTP?1") -> (6:w800:errorcluster)  [unwired: 3 in, 1 out]
                                n680 = GPIB Read(0:w794, 1:3200, 3:w800) -> (5:w798:string)  [unwired: 2 in, 2 out]
                                n681 = Fract/Exp String To Number(string=w798) -> (number=w797:dbl)  [unwired: 3 in, 1 out]
                                n682 = Build Array (concatenate)(w802, w797) -> (w801:dbl[])
                              }
                            }
                            n683 = property on="data" class="Arr (strict)"("Value"=w792) -> ()  [unwired: 2 in, 2 out]
                          }
                          frame #3 {
                            # "check if out-of-phase\nsignal on lock-in 2 \nis to be measured"
                            n684 = property on="data" class="Arr (strict)"() -> ("Value"=w804:dbl[])  [unwired: 2 in, 2 out]
                            n685 = local read "SR830 2 oop"() -> (w803:bool)
                            n686 = case shown="True" w803 {
                              tunnel: w804 -> [w806 w815]
                              tunnel: [w806 w814] -> w805
                              frame False {
                                # "we are not measuring out of phase signal on lock-in 2 (SR830_2_oop)"
                              }
                              frame True {
                                # "we are  measuring lock-in 2, out of phase (SR830_2_oop)"
                                n687 = local read "SR830 2 addr"() -> (w808:u8)
                                n688 = Number To Decimal String(number=w808) -> (decimal integer string=w807:string)  [unwired: 1 in]
                                n689 = GPIB Write(0:w807, 1:"OUTP?2") -> (6:w813:errorcluster)  [unwired: 3 in, 1 out]
                                n690 = GPIB Read(0:w807, 1:3200, 3:w813) -> (5:w811:string)  [unwired: 2 in, 2 out]
                                n691 = Fract/Exp String To Number(string=w811) -> (number=w810:dbl)  [unwired: 3 in, 1 out]
                                n692 = Build Array (concatenate)(w815, w810) -> (w814:dbl[])
                              }
                            }
                            n693 = property on="data" class="Arr (strict)"("Value"=w805) -> ()  [unwired: 2 in, 2 out]
                          }
                          frame #4 {
                            # "check if in-phase\nsignal on lock-in 3 \nis to be measured"
                            n694 = property on="data" class="Arr (strict)"() -> ("Value"=w817:dbl[])  [unwired: 2 in, 2 out]
                            n695 = local read "SR830 3 ip"() -> (w816:bool)
                            n696 = case shown="True" w816 {
                              tunnel: w817 -> [w819 w828]
                              tunnel: [w819 w827] -> w818
                              frame False {
                                # "we are not measuring in phase signal on lock-in 3 (SR830_3_ip)"
                              }
                              frame True {
                                # "we are  measuring lock-in 3, in phase (SR830_3_ip)"
                                n697 = local read "SR830 3 addr"() -> (w821:u8)
                                n698 = Number To Decimal String(number=w821) -> (decimal integer string=w820:string)  [unwired: 1 in]
                                n699 = GPIB Write(0:w820, 1:"OUTP?1") -> (6:w826:errorcluster)  [unwired: 3 in, 1 out]
                                n700 = GPIB Read(0:w820, 1:3200, 3:w826) -> (5:w824:string)  [unwired: 2 in, 2 out]
                                n701 = Fract/Exp String To Number(string=w824) -> (number=w823:dbl)  [unwired: 3 in, 1 out]
                                n702 = Build Array (concatenate)(w828, w823) -> (w827:dbl[])
                              }
                            }
                            n703 = property on="data" class="Arr (strict)"("Value"=w818) -> ()  [unwired: 2 in, 2 out]
                          }
                          frame #5 {
                            # "check if out-of-phase\nsignal on lock-in 3 \nis to be measured"
                            n704 = property on="data" class="Arr (strict)"() -> ("Value"=w830:dbl[])  [unwired: 2 in, 2 out]
                            n705 = local read "SR830 3 oop"() -> (w829:bool)
                            n706 = case shown="True" w829 {
                              tunnel: w830 -> [w832 w841]
                              tunnel: [w832 w840] -> w831
                              frame False {
                                # "we are not measuring out of phase signal on lock-in 3 (SR830_3_oop)"
                              }
                              frame True {
                                # "we are  measuring lock-in 3, out of phase (SR830_3_oop)"
                                n707 = local read "SR830 3 addr"() -> (w834:u8)
                                n708 = Number To Decimal String(number=w834) -> (decimal integer string=w833:string)  [unwired: 1 in]
                                n709 = GPIB Write(0:w833, 1:"OUTP?2") -> (6:w839:errorcluster)  [unwired: 3 in, 1 out]
                                n710 = GPIB Read(0:w833, 1:3200, 3:w839) -> (5:w837:string)  [unwired: 2 in, 2 out]
                                n711 = Fract/Exp String To Number(string=w837) -> (number=w836:dbl)  [unwired: 3 in, 1 out]
                                n712 = Build Array (concatenate)(w841, w836) -> (w840:dbl[])
                              }
                            }
                            n713 = property on="data" class="Arr (strict)"("Value"=w831) -> ()  [unwired: 2 in, 2 out]
                          }
                          frame #6 {
                            # "check if in-phase\nsignal on lock-in 4 \nis to be measured"
                            n714 = property on="data" class="Arr (strict)"() -> ("Value"=w843:dbl[])  [unwired: 2 in, 2 out]
                            n715 = local read "SR830 4 ip"() -> (w842:bool)
                            n716 = case shown="True" w842 {
                              tunnel: w843 -> [w845 w854]
                              tunnel: [w845 w853] -> w844
                              frame False {
                                # "we are not measuring in phase signal on lock-in 4 (SR830_4_ip)"
                              }
                              frame True {
                                # "we are  measuring lock-in 4, in phase (SR830_4_ip)"
                                n717 = local read "SR830 4 addr"() -> (w847:u8)
                                n718 = Number To Decimal String(number=w847) -> (decimal integer string=w846:string)  [unwired: 1 in]
                                n719 = GPIB Write(0:w846, 1:"OUTP?1") -> (6:w852:errorcluster)  [unwired: 3 in, 1 out]
                                n720 = GPIB Read(0:w846, 1:3200, 3:w852) -> (5:w850:string)  [unwired: 2 in, 2 out]
                                n721 = Fract/Exp String To Number(string=w850) -> (number=w849:dbl)  [unwired: 3 in, 1 out]
                                n722 = Build Array (concatenate)(w854, w849) -> (w853:dbl[])
                              }
                            }
                            n723 = property on="data" class="Arr (strict)"("Value"=w844) -> ()  [unwired: 2 in, 2 out]
                          }
                          frame #7 {
                            # "check if out-of-phase\nsignal on lock-in 4 \nis to be measured"
                            n724 = property on="data" class="Arr (strict)"() -> ("Value"=w856:dbl[])  [unwired: 2 in, 2 out]
                            n725 = local read "SR830 4 oop"() -> (w855:bool)
                            n726 = case shown="True" w855 {
                              tunnel: w856 -> [w858 w867]
                              tunnel: [w858 w866] -> w857
                              frame False {
                                # "we are not measuring out of phase signal on lock-in 4 (SR830_4_oop)"
                              }
                              frame True {
                                # "we are  measuring lock-in 4, out of phase (SR830_4_oop)"
                                n727 = local read "SR830 4 addr"() -> (w860:u8)
                                n728 = Number To Decimal String(number=w860) -> (decimal integer string=w859:string)  [unwired: 1 in]
                                n729 = GPIB Write(0:w859, 1:"OUTP?2") -> (6:w865:errorcluster)  [unwired: 3 in, 1 out]
                                n730 = GPIB Read(0:w859, 1:3200, 3:w865) -> (5:w863:string)  [unwired: 2 in, 2 out]
                                n731 = Fract/Exp String To Number(string=w863) -> (number=w862:dbl)  [unwired: 3 in, 1 out]
                                n732 = Build Array (concatenate)(w867, w862) -> (w866:dbl[])
                              }
                            }
                            n733 = property on="data" class="Arr (strict)"("Value"=w857) -> ()  [unwired: 2 in, 2 out]
                          }
                          frame #8 {
                            # "check if voltage \non 2400 SouceMeter 1\nis to be measured"
                            n734 = property on="data" class="Arr (strict)"() -> ("Value"=w869:dbl[])  [unwired: 2 in, 2 out]
                            n735 = local read "2400 1 meas v"() -> (w868:bool)
                            n736 = case shown="True" w868 {
                              tunnel: w869 -> [w871 w882]
                              tunnel: [w871 w881] -> w870
                              frame False {
                                # "we are not measuring 2400 1, voltage (2400_1_v)"
                              }
                              frame True {
                                # "we are  measuring 2400 1, voltage (2400_1_v)"
                                n737 = local read "2400 1 addr"() -> (w876:u8)
                                n738 = Number To Decimal String(number=w876) -> (decimal integer string=w875:string)  [unwired: 1 in]
                                n739 = GPIB Write(0:w875, 1:":READ?") -> (6:w880:errorcluster)  [unwired: 3 in, 1 out]
                                n740 = GPIB Read(0:w875, 1:3200, 3:w880) -> (5:w873:string)  [unwired: 2 in, 2 out]
                                n741 = String Subset(string=w873, length (rest)=13) -> (substring=w872:string)  [unwired: 1 in]
                                n742 = Fract/Exp String To Number(string=w872) -> (number=w878:dbl)  [unwired: 3 in, 1 out]
                                n743 = Build Array (concatenate)(w882, w878) -> (w881:dbl[])
                              }
                            }
                            n744 = property on="data" class="Arr (strict)"("Value"=w870) -> ()  [unwired: 2 in, 2 out]
                          }
                          frame #9 {
                            # "check if current \non 2400 SouceMeter 1\nis to be measured"
                            n745 = property on="data" class="Arr (strict)"() -> ("Value"=w884:dbl[])  [unwired: 2 in, 2 out]
                            n746 = local read "2400 1 meas i"() -> (w883:bool)
                            n747 = case shown="True" w883 {
                              tunnel: w884 -> [w886 w898]
                              tunnel: [w886 w897] -> w885
                              frame False {
                                # "we are not measuring 2400 1, current (2400_1_i)"
                              }
                              frame True {
                                # "we are  measuring 2400 1, current (2400_1_i)"
                                n748 = local read "2400 1 addr"() -> (w892:u8)
                                n749 = Number To Decimal String(number=w892) -> (decimal integer string=w891:string)  [unwired: 1 in]
                                n750 = GPIB Write(0:w891, 1:":READ?") -> (6:w896:errorcluster)  [unwired: 3 in, 1 out]
                                n751 = GPIB Read(0:w891, 1:3200, 3:w896) -> (5:w889:string)  [unwired: 2 in, 2 out]
                                n752 = String Subset(string=w889, offset (0)=14, length (rest)=13) -> (substring=w888:string)
                                n753 = Fract/Exp String To Number(string=w888) -> (number=w894:dbl)  [unwired: 3 in, 1 out]
                                n754 = Build Array (concatenate)(w898, w894) -> (w897:dbl[])
                              }
                            }
                            n755 = property on="data" class="Arr (strict)"("Value"=w885) -> ()  [unwired: 2 in, 2 out]
                          }
                          frame #10 {
                            # "check if voltage \non 2400 SouceMeter 2\nis to be measured"
                            n756 = property on="data" class="Arr (strict)"() -> ("Value"=w900:dbl[])  [unwired: 2 in, 2 out]
                            n757 = local read "2400 2 meas v"() -> (w899:bool)
                            n758 = case shown="True" w899 {
                              tunnel: w900 -> [w902 w913]
                              tunnel: [w902 w912] -> w901
                              frame False {
                                # "we are not measuring 2400 2, voltage (2400_2_v)"
                              }
                              frame True {
                                # "we are  measuring 2400 2, voltage (2400_2_v)"
                                n759 = local read "2400 2 addr"() -> (w907:u8)
                                n760 = Number To Decimal String(number=w907) -> (decimal integer string=w906:string)  [unwired: 1 in]
                                n761 = GPIB Write(0:w906, 1:":READ?") -> (6:w911:errorcluster)  [unwired: 3 in, 1 out]
                                n762 = GPIB Read(0:w906, 1:3200, 3:w911) -> (5:w904:string)  [unwired: 2 in, 2 out]
                                n763 = String Subset(string=w904, length (rest)=13) -> (substring=w903:string)  [unwired: 1 in]
                                n764 = Fract/Exp String To Number(string=w903) -> (number=w909:dbl)  [unwired: 3 in, 1 out]
                                n765 = Build Array (concatenate)(w913, w909) -> (w912:dbl[])
                              }
                            }
                            n766 = property on="data" class="Arr (strict)"("Value"=w901) -> ()  [unwired: 2 in, 2 out]
                          }
                          frame #11 {
                            # "check if current \non 2400 SouceMeter 2\nis to be measured"
                            n767 = property on="data" class="Arr (strict)"() -> ("Value"=w915:dbl[])  [unwired: 2 in, 2 out]
                            n768 = local read "2400 2 meas i"() -> (w914:bool)
                            n769 = case shown="True" w914 {
                              tunnel: w915 -> [w917 w929]
                              tunnel: [w917 w928] -> w916
                              frame False {
                                # "we are not measuring 2400 2, current (2400_2_i)"
                              }
                              frame True {
                                # "we are  measuring 2400 2, current (2400_2_i)"
                                n770 = local read "2400 2 addr"() -> (w923:u8)
                                n771 = Number To Decimal String(number=w923) -> (decimal integer string=w922:string)  [unwired: 1 in]
                                n772 = GPIB Write(0:w922, 1:":READ?") -> (6:w927:errorcluster)  [unwired: 3 in, 1 out]
                                n773 = GPIB Read(0:w922, 1:3200, 3:w927) -> (5:w920:string)  [unwired: 2 in, 2 out]
                                n774 = String Subset(string=w920, offset (0)=14, length (rest)=13) -> (substring=w919:string)
                                n775 = Fract/Exp String To Number(string=w919) -> (number=w925:dbl)  [unwired: 3 in, 1 out]
                                n776 = Build Array (concatenate)(w929, w925) -> (w928:dbl[])
                              }
                            }
                            n777 = property on="data" class="Arr (strict)"("Value"=w916) -> ()  [unwired: 2 in, 2 out]
                          }
